vi "Do.vi"(6 "Input":variant, 8 "error in":errorcluster, 9 "Self Enqueuer":refnum<class "Message Enqueuer.lvclass">, 10 "Series Enqueuer":refnum<class "Message Enqueuer.lvclass">, 11 "Sample PI Control in":refnum<class "Sample PI Control.lvclass">) -> (0 "error out":errorcluster, 3 "Sample PI Control out":refnum<class "Sample PI Control.lvclass">)   [LabVIEW 2023, in "Sample PI Control.lvclass"]
uses:
  Sample PI Control.lvclass
  Sample PI Control.lvclass/Sample PI Control.ctl
  Task/Task Base/Task Base.lvclass
  <vilib>/addons/control/pid/NI_PID_pid.lvlib
  Measure and Stimulus Subsystems/Measure and Stimulus Subsystems.lvclass
  Series/ISeries Actor/ISeries Actor Messages/Point Data Updated Msg/Point Data Updated Msg.lvclass
  <vilib>/addons/control/pid/pid.llb/PID (DBL).vi
  <vilib>/ActorFramework/Message Enqueuer/Message Enqueuer.lvclass
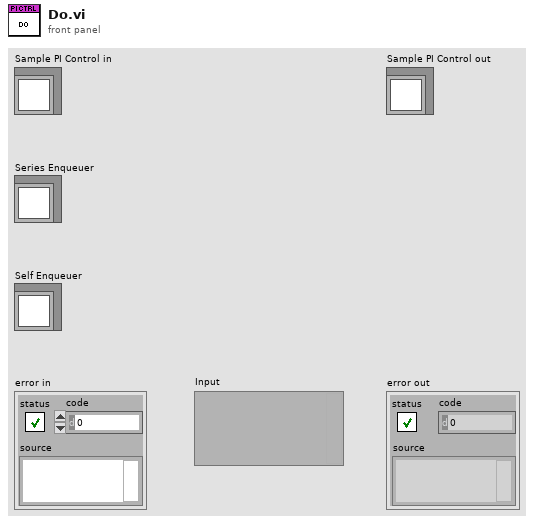
[diagram p1: front panel]
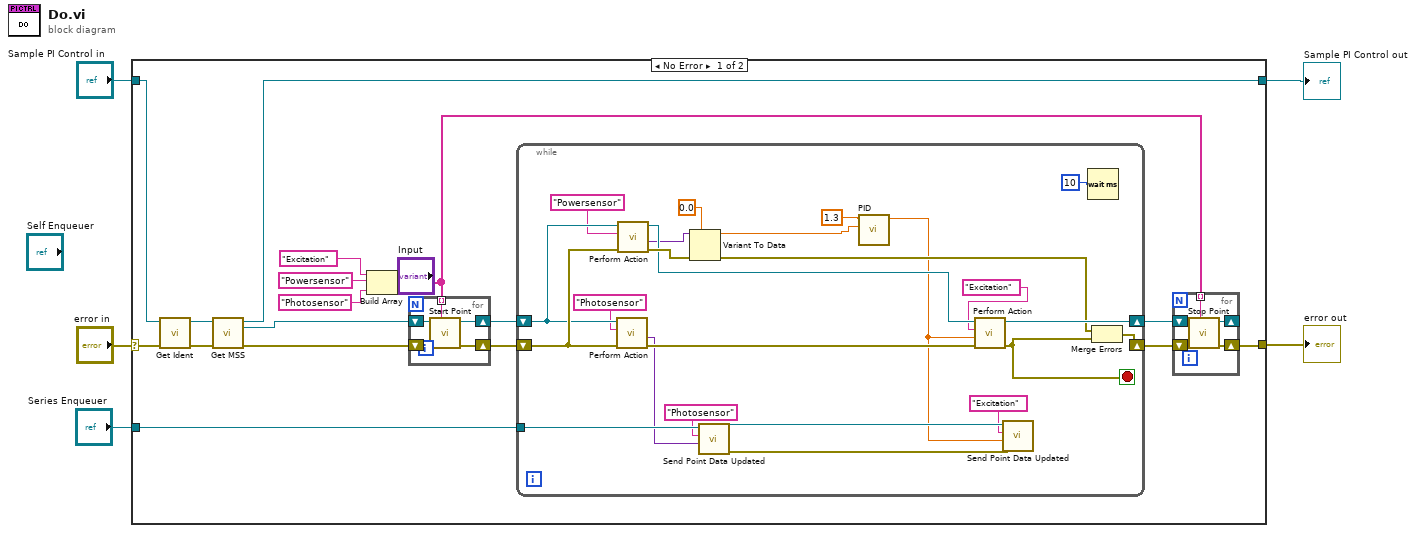
[diagram p0: block diagram]
diagram:
  n1 = case shown="No Error" "error in" {
    selector: "error in" -> [w19 w58]
    tunnel: [w15 w58] -> w4
    tunnel: [w10 w57] -> w2
    tunnel: "Sample PI Control in" -> [w7 w57]
    tunnel: "Series Enqueuer" -> [w9 _]
    frame No Error {
      n2 = call "Get Ident.vi"("error in (no error)"=w19, "Task Base in"=w7) -> ("error out"=w8:errorcluster, "Task Base out"=w6:refnum<class "Sample PI Control.lvclass">)  [unwired: 7 in, 1 out]
      n3 = call "Get MSS.vi"("error in (no error)"=w8, "Task Base in"=w6) -> ("error out"=w18:errorcluster, "MSS"=w17:refnum<class "Measure and Stimulus Subsystems.lvclass">, "Task Base out"=w10:refnum<class "Sample PI Control.lvclass">)  [unwired: 7 in]
      n4 = Build Array("Excitation" ("Target Ident"), "Powersensor" ("Target Identifier"), "Photosensor" ("Target Identifier")) -> (w11:string[])
      n5 = for {
        shift-right: [w27] -> w22
        shift-left: w18 -> [w25]
        shift-right: [w26] -> w21
        shift-left: w17 -> [w24]
        tunnel: w11 -> [w23] mode=indexing
        n6 = call "Start Point.vi"("Point Ident"=w23, "error in"=w25, "MSS in"=w24) -> ("error out"=w27:errorcluster, "MSS out"=w26:refnum<class "Measure and Stimulus Subsystems.lvclass">)  [unwired: 7 in]
      }
      n7 = while {
        shift-right: [w43] -> w20
        shift-left: w22 -> [w48]
        shift-right: [w49] -> w16
        shift-left: w21 -> [w47]
        tunnel: w9 -> [w38]
        stop <- w41 stop-if-true
        n8 = call "Perform Action.vi"("error in"=w48, "Point Ident"="Photosensor" ("Target Identifier"), "MSS in"=w47) -> ("error out"=w39:errorcluster, "Output"=w32:variant)  [unwired: 5 in, 2 out]
        n9 = call "Perform Action.vi"("error in"=w48, "Point Ident"="Powersensor" ("Target Identifier"), "MSS in"=w47) -> ("error out"=w51:errorcluster, "Output"=w29:variant, "MSS out"=w44:refnum<class "Measure and Stimulus Subsystems.lvclass">)  [unwired: 5 in, 1 out]
        n10 = Variant To Data(error in=w51, type=0.0, Variant=w29) -> (data=w45:dbl, error out=w42:errorcluster)
        n11 = call "Send Point Data Updated.vi"("Data"=w32, "Task-Point Ident"="Photosensor" ("Target Identifier"), "Message Enqueuer"=w38) -> ("error out"=w36:errorcluster, "Message Enqueuer out"=w35:refnum<class "Message Enqueuer.lvclass">)  [unwired: 7 in]
        n12 = call-poly <vilib>:"PID.vi"("process variable"=w45, "setpoint"=1.3) -> ("output"=w31:dbl)  [unwired: 8 in, 1 out]
        n13 = call "Perform Action.vi"("error in"=w39, "Input"=w31, "Point Ident"="Excitation" ("Target Ident"), "MSS in"=w44) -> ("error out"=w41:errorcluster, "MSS out"=w49:refnum<class "Measure and Stimulus Subsystems.lvclass">)  [unwired: 4 in, 2 out]
        n14 = call "Send Point Data Updated.vi"("error in (no error)"=w36, "Data"=w31, "Task-Point Ident"="Excitation" ("Target Ident"), "Message Enqueuer"=w35) -> ()  [unwired: 6 in, 2 out]
        n15 = Wait (ms)(milliseconds to wait=u32 10) -> ()  [unwired: 1 out]
        n16 = Merge Errors(w42, w41) -> (w43:errorcluster)
      }
      n17 = for {
        shift-right: [w54] -> w15
        shift-left: w20 -> [w56]
        tunnel: w11 -> [w52] mode=indexing
        shift-right: [w53] -> _
        shift-left: w16 -> [w55]
        n18 = call "Stop Point.vi"("Point Ident"=w52, "error in"=w56, "MSS in"=w55) -> ("error out"=w54:errorcluster, "MSS out"=w53:refnum<class "Measure and Stimulus Subsystems.lvclass">)  [unwired: 7 in]
      }
    }
    frame Error {
    }
  }
  "error out" <- w4
  "Sample PI Control out" <- w2
